vi "Main.vi"() -> ()   [LabVIEW 2014]
panel:
  in  "Stop Button":bool
  in  "Media Stop Button":bool
  in  "Couleur Auto":bool
  in  "Couleur manuelle":bool
  in  "Adresse du serveur":string="192.168.1.200"
  in  "Couleur manuelle":u32(colorbox)=6618880
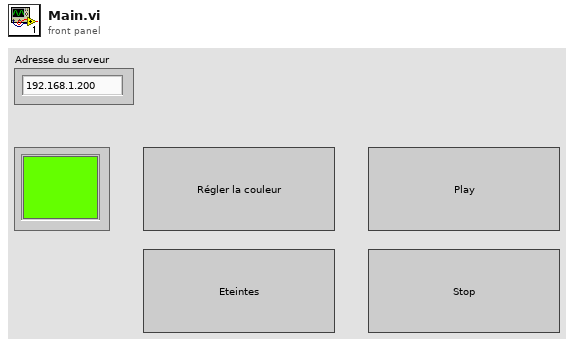
[diagram p1: front panel]
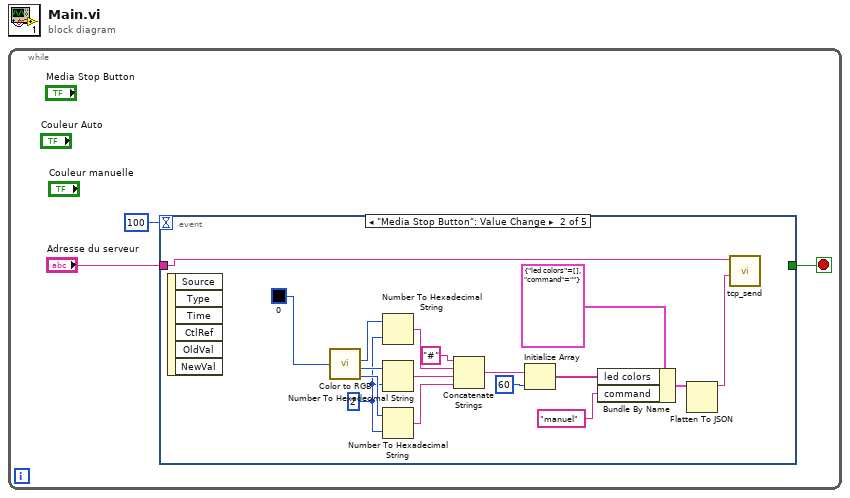
[diagram p0: block diagram]
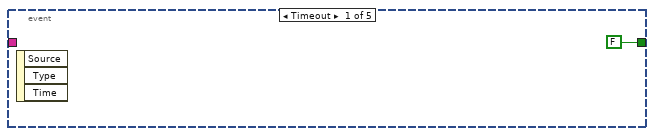
[diagram p2: hidden frame]
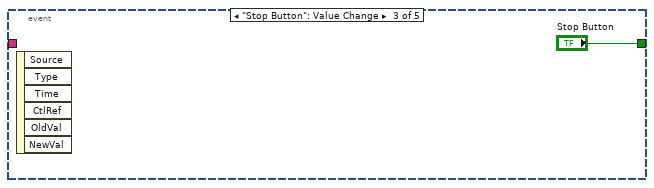
[diagram p3: hidden frame]
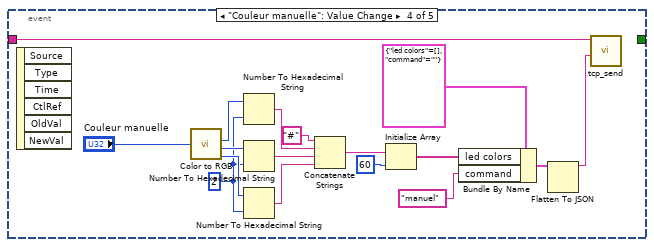
[diagram p4: hidden frame]
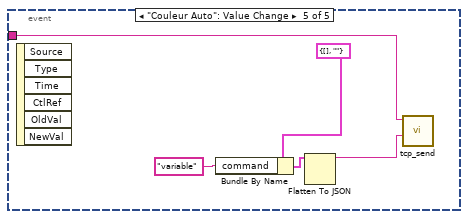
[diagram p5: hidden frame]
diagram:
  n1 = while {
    stop <- w2 stop-if-true
    n2 = event shown="[1] \"Media Stop Button\": Value Change" {
      selector: _ -> [_ _ _ _ _]
      dyn-events: _ -> [_ _ _ _ _]
      timeout: 100 -> [_ _ _ _ _]
      tunnel: [FALSE _ "Stop Button" _ _] -> w2
      tunnel: "Adresse du serveur" -> [_ w6 _ w23 w40]
      event Timeout {
        n3 = event-data() -> ()  [unwired: 1 in, 3 out]
      }
      event "Media Stop Button": Value Change {
        w12 = i16 2 ("width (-)")
        n4 = event-data() -> ()  [unwired: 1 in, 6 out]
        n5 = call <vilib>:"Color to RGB.vi"("Color"=u32 0) -> ("R"=w11:u8, "G"=w13:u8, "B"=w14:u8)  [unwired: 1 out]
        n6 = Number To Hexadecimal String(1:w12, 2:w11) -> (0:w15:string)
        n7 = Number To Hexadecimal String(1:w12, 2:w13) -> (0:w16:string)
        n8 = Number To Hexadecimal String(1:w12, 2:w14) -> (0:w17:string)
        n9 = Concatenate Strings("#", w15, w16, w17) -> (w19:string)
        n10 = Initialize Array(w19, 60 ("dimension size")) -> (w21:string[])
        n11 = Bundle By Name(cluster=cluster{"led colors":string[], "command":string} {"led colors"=[], "command"=""}, "led colors"=w21, "command"="manuel") -> (w9:cluster{"led colors":string[], "command":string})
        n12 = Flatten To JSON(anything=w9) -> (JSON string=w7:string)  [unwired: 2 in, 1 out]
        n13 = call "tcp_send.vi"("Message JSON"=w7, "Adresse du serveur"=w6) -> ()  [unwired: 10 in]
      }
      event "Stop Button": Value Change {
        n14 = event-data() -> ()  [unwired: 1 in, 6 out]
      }
      event "Couleur manuelle": Value Change {
        w30 = i16 2 ("width (-)")
        n15 = event-data() -> ()  [unwired: 1 in, 6 out]
        n16 = call <vilib>:"Color to RGB.vi"("Color"="Couleur manuelle") -> ("R"=w29:u8, "G"=w31:u8, "B"=w32:u8)  [unwired: 1 out]
        n17 = Number To Hexadecimal String(1:w30, 2:w29) -> (0:w33:string)
        n18 = Number To Hexadecimal String(1:w30, 2:w31) -> (0:w34:string)
        n19 = Number To Hexadecimal String(1:w30, 2:w32) -> (0:w35:string)
        n20 = Concatenate Strings("#", w33, w34, w35) -> (w37:string)
        n21 = Initialize Array(w37, 60 ("dimension size")) -> (w39:string[])
        n22 = Bundle By Name(cluster=cluster{"led colors":string[], "command":string} {"led colors"=[], "command"=""}, "led colors"=w39, "command"="manuel") -> (w26:cluster{"led colors":string[], "command":string})
        n23 = Flatten To JSON(anything=w26) -> (JSON string=w24:string)  [unwired: 2 in, 1 out]
        n24 = call "tcp_send.vi"("Message JSON"=w24, "Adresse du serveur"=w23) -> ()  [unwired: 10 in]
      }
      event "Couleur Auto": Value Change {
        n25 = event-data() -> ()  [unwired: 1 in, 6 out]
        n26 = Bundle By Name(cluster=cluster{"led colors":string[], "command":string} {"led colors"=[], "command"=""}, "command"="variable") -> (w44:cluster{"led colors":string[], "command":string})
        n27 = Flatten To JSON(anything=w44) -> (JSON string=w41:string)  [unwired: 2 in, 1 out]
        n28 = call "tcp_send.vi"("Message JSON"=w41, "Adresse du serveur"=w40) -> ()  [unwired: 10 in]
      }
    }
  }
